vi "ESN_RiffleTrainingPairs.vi"(11 "Input output pairs":cluster{"Input":dbl[], "Output":dbl[]}[](array[cluster])) -> (3 "Input output pairs":cluster{"Input":dbl[], "Output":dbl[]}[](array[cluster]))   [LabVIEW 2017]
uses:
  <vilib>/Analysis/1siggen.llb/Ramp Pattern by Samples.vi
  <vilib>/Analysis/1siggen.llb/Riffle Array (DBL) (obs 2012).vi
  <vilib>/Analysis/NI_AALBase.lvlib
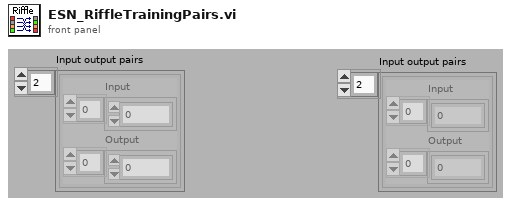
[diagram p1: front panel]
types:
  T1 = cluster{dbl, "Input output pairs":cluster{"Input":dbl[], "Output":dbl[]}}
  T2 = cluster{dbl, "Input output pairs":cluster{"Input":dbl[], "Output":dbl[]}}[]
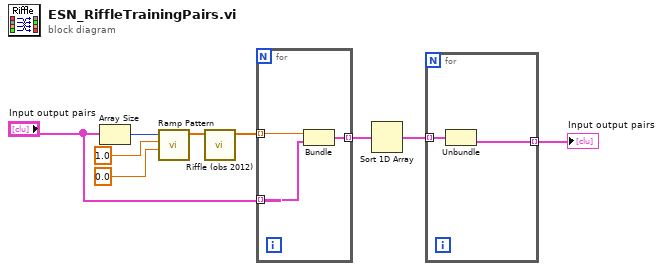
[diagram p0: block diagram]
diagram:
  n1 = Array Size(array="Input output pairs") -> (size(s)=w9:i32)
  n2 = call-poly <vilib>:"Ramp Pattern.vi"("start"=0.0, "end"=1.0, "samples"=w9) -> ("Ramp Pattern"=w6:dbl[])  [unwired: 7 in, 1 out]
  n3 = call-poly <vilib>:"Riffle (obs 2012).vi"("X"=w6) -> ("Riffled {X}"=w4:dbl[])  [unwired: 8 in, 2 out]
  n4 = for {
    tunnel: "Input output pairs" -> [w11] mode=indexing
    tunnel: w4 -> [w12] mode=indexing
    tunnel: [w10] -> w3 mode=indexing
    n5 = Bundle(w12, "Input output pairs"=w11) -> (w10:T1)  [unwired: 1 in]
  }
  n6 = Sort 1D Array(array=w3) -> (sorted array=w2:T2)
  n7 = for {
    tunnel: w2 -> [w14] mode=indexing
    tunnel: [w13] -> w1 mode=indexing
    n8 = Unbundle(w14) -> ("Input output pairs"=w13:cluster{"Input":dbl[], "Output":dbl[]})  [unwired: 1 out]
  }
  "Input output pairs" <- w1
